vi "IR Transmit Raw.vi"(0 "Arduino Resource":T2={"VISA resource"="", "Board Type"=enum."Arduino Uno", "Connection Type"=enum."USB / Serial", "Bytes Per Packet (15)"=15}, 5 "IR Type":T1, 7 "Data":u32, 9 "Number Of Bits (32 Max)":u8=32, 11 "Error In":errorcluster) -> (4 "Arduino Resource":T2={"VISA resource"="", "Board Type"=enum."Arduino Uno", "Connection Type"=enum."USB / Serial", "Bytes Per Packet (15)"=15}, 15 "Error Out":errorcluster)   [LabVIEW 2011, in "LabVIEW Interface for ChipKit.lvlib"]
uses:
  LabVIEW Interface for ChipKit.lvlib
  Private/Type Defs/Chipkit Resource.ctl
  Private/Type Defs/Board Type.ctl
  Private/Type Defs/IR Type.ctl
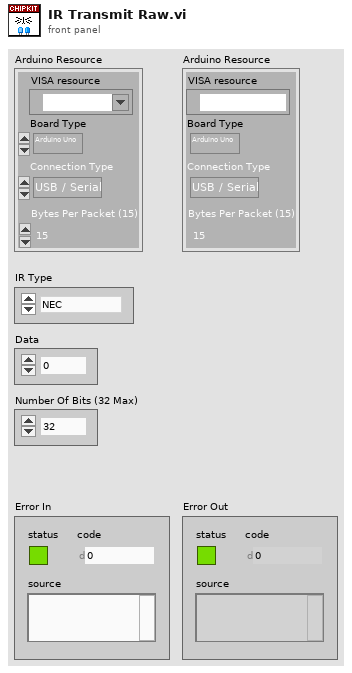
[diagram p1: front panel]
types:
  T1 = typedef "LabVIEW Interface for ChipKit.lvlib/IR Type.ctl" = enum8{"NEC", "Sony", "RC5", "RC6"}
  T2 = typedef "LabVIEW Interface for ChipKit.lvlib/Chipkit Resource.ctl" = cluster{"VISA resource":refnum<visa-resource-name>, "Board Type":T3, "Connection Type":enum8{"USB / Serial"}, "Bytes Per Packet (15)":u8}
  T3 = typedef "LabVIEW Interface for ChipKit.lvlib/Board Type.ctl" = enum16{"Arduino Uno", "Dimuelanove w/Atmega 328", "Mega 2560", "Chipkit Uno32", "Chipkit Max32"}
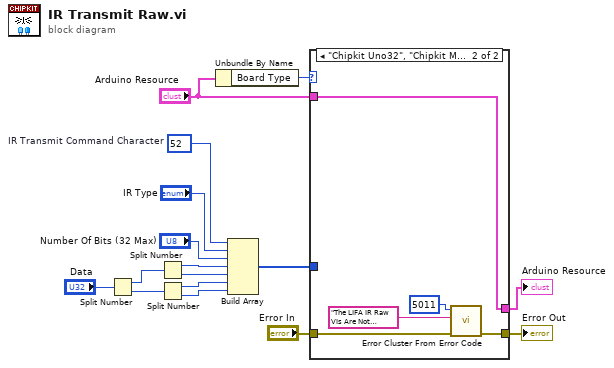
[diagram p0: block diagram]
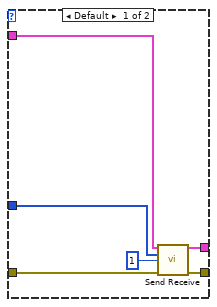
[diagram p2: hidden frame]
diagram:
  w15 = u8 52  # IR Transmit Command Character
  n1 = Split Number(x="Data") -> (hi(x)=w11:u16, lo(x)=w12:u16)
  n2 = Split Number(x=w11) -> (hi(x)=w10:u8, lo(x)=w9:u8)
  n3 = Split Number(x=w12) -> (hi(x)=w8:u8, lo(x)=w7:u8)
  n4 = Unbundle By Name("Arduino Resource") -> ("Board Type"=w1:T3)
  n5 = Build Array(w15, "IR Type", "Number Of Bits (32 Max)", w10, w9, w8, w7) -> (w5:u8[])
  n6 = case shown="\"Chipkit Uno32\", \"Chipkit Max32\"" w1 {
    tunnel: "Error In" -> [w21 w25]
    tunnel: [w20 w24] -> w3
    tunnel: w5 -> [w19 _]
    tunnel: [w18 w23] -> w4
    tunnel: "Arduino Resource" -> [w17 w23]
    frame Default {
      n7 = call "Send Receive.vi"("Arduino Resource"=w17, "Data"=w19, "Bytes To Read (0)"=u8 1, "error in"=w21) -> ("Arduino Resource"=w18:T2, "error out"=w20:errorcluster)  [unwired: 9 in, 1 out]
    }
    frame "Chipkit Uno32", "Chipkit Max32" {
      n8 = call <vilib>:"Error Cluster From Error Code.vi"("error in (no error)"=w25, "error message (\"\")"="The LIFA IR Raw VIs Are Not Supported On Chipkit Targets." ("source"), "error code (0)"=5011) -> ("error out"=w24:errorcluster)  [unwired: 6 in]
    }
  }
  "Arduino Resource" <- w4
  "Error Out" <- w3
